vi "ColorCellBG.vi"(6 "Cell Position":T1, 8 "error in (no error)":errorcluster, 9 "Table CtlRef In":refnum<vi>, 10 "Value":string, 11 "MenuCol in":refnum<class "MenuCol.lvclass">) -> (0 "error out":errorcluster, 1 "Table CtlRef Out":refnum<vi>, 3 "MenuCol out":refnum<class "MenuCol.lvclass">)   [LabVIEW 2013, in "MenuCol.lvclass"]
uses:
  MenuCol.lvclass
  <vilib>/Utility/miscctls.llb/LVRowAndColumnTypeDef.ctl
  Column/Column.lvclass/Column.ctl
  Globals/DisabledColorGlobal.vi
  Column/Column.lvclass
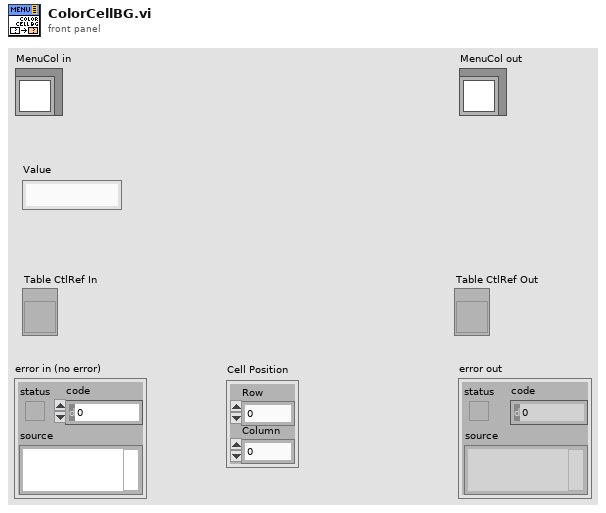
[diagram p1: front panel]
types:
  T1 = typedef "LVRowAndColumnTypeDef.ctl" = cluster{"Row":i32, "Column":i32}
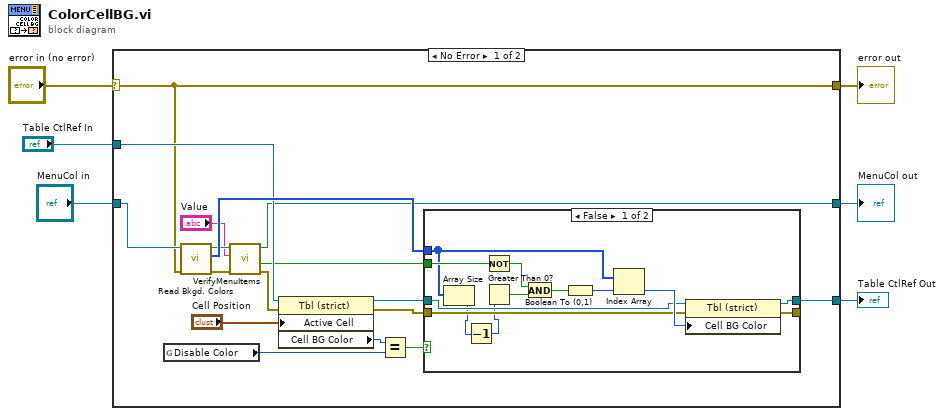
[diagram p0: block diagram]
diagram:
  n1 = case shown="No Error" "error in (no error)" {
    selector: "error in (no error)" -> [w9 w41]
    tunnel: [w9 w41] -> w5
    tunnel: [w13 w40] -> w3
    tunnel: "MenuCol in" -> [w10 w40]
    tunnel: "Table CtlRef In" -> [w15 w39]
    tunnel: [w17 w39] -> w1
    frame No Error {
      n2 = global read "DisabledColorGlobal.vi" "Disable Color"() -> (w19:u32)
      n3 = call "Read Bkgd. Colors.vi"("error in (no error)"=w9, "Column in"=w10) -> ("error out"=w12:errorcluster, "Bkgd. Colors"=w18:u32[], "Column out"=w14:refnum<class "MenuCol.lvclass">)  [unwired: 7 in]
      n4 = call-dynamic "VerifyMenuItems.vi"("error in (no error)"=w12, "Menu Item In"="Value", "MenuCol in"=w14) -> ("error out"=w11:errorcluster, "Valid Menu Item"=w7:bool, "MenuCol out"=w13:refnum<class "MenuCol.lvclass">)  [unwired: 5 in, 1 out]
      n5 = property class="Tbl (strict)"(reference=w15, error in=w11, "Active Cell"="Cell Position") -> (reference out=w21:refnum<vi>, error out=w22:errorcluster, "Cell BG Color"=w20:u32)
      n6 = Equal?(x=w20, y=w19) -> (x = y?=w23:bool)
      n7 = case shown="False" w23 {
        tunnel: w18 -> [w30 _]
        tunnel: [w35 w37] -> _
        tunnel: [w34 w38] -> w17
        tunnel: w21 -> [w33 w38]
        tunnel: w22 -> [w32 w37]
        tunnel: w7 -> [w31 _]
        frame False {
          n8 = Array Size(array=w30) -> (size(s)=w25:i32)
          n9 = Decrement(x=w25) -> (x-1=w24:i32)
          n10 = Not(x=w31) -> (.not. x?=w28:bool)
          n11 = Greater Than 0?(x=w24) -> (x > 0?=w29:bool)
          n12 = And(x=w28, y=w29) -> (x .and. y?=w27:bool)
          n13 = Boolean To (0,1)(Boolean=w27) -> (0, 1=w26:i16)
          n14 = Index Array(array=w30, index=w26) -> (element=w36:u32)
          n15 = property class="Tbl (strict)"(reference=w33, error in=w32, "Cell BG Color"=w36) -> (reference out=w34:refnum<vi>, error out=w35:errorcluster)
        }
        frame True {
        }
      }
    }
    frame Error {
    }
  }
  "error out" <- w5
  "MenuCol out" <- w3
  "Table CtlRef Out" <- w1
